vi "Teleop With Vision.vi"(10 "Match Info":T1={"Autonomous Elapsed Seconds"=0.0, "TeleOp Elapsed Seconds"=0.0, "Disabled Elapsed Seconds"=0.0, "Visited Autonomous"=FALSE, "Visited TeleOp"=FALSE, "Visited Disabled"=FALSE, "Autonomous Settings"={"Autonomous Style"=enum."Independent", "VI Refnum"=refnum}}, 11 "Call Context":T2=enum."Execute") -> ()   [LabVIEW 2012]
doc: "This VI is called for each TeleOp packet received from the DS where the robot is not disabled. It is often used to read from the joysticks and update I/O or to update setpoints for timed control loops. It should complete and return within 20 milliseconds or it may miss DS packets."
uses:
  <vilib>/Rock Robotics/WPI/DriverStation/WPI_DriverStationDerivedRobotMode.ctl
  <vilib>/Rock Robotics/WPI/DriverStation/WPI_DriverStationMatch Info.ctl
  Robot Global Data.vi
  <vilib>/Rock Robotics/WPI/RobotDrive/WPI_RobotDriveMecanumDrive_Cartesian.vi
  <vilib>/Rock Robotics/WPI/Joystick/WPI_JoystickGetSetRefNum.vi
  <vilib>/Rock Robotics/WPI/RobotDrive/WPI_RobotDriveGetSetRefNum.vi
panel:
  in  "Rotation Mult":dbl=0.8
  in  "Joystick Mult Slow":dbl=0.5
  in  "Joystick Mult":dbl=1.0
  in  "Rest Speed r/s":dbl=15.0 min=0.0 max=0.7 step=0.05
  out "Angle":dbl(knob)=359.9532640347576 scale=0.0..360.0
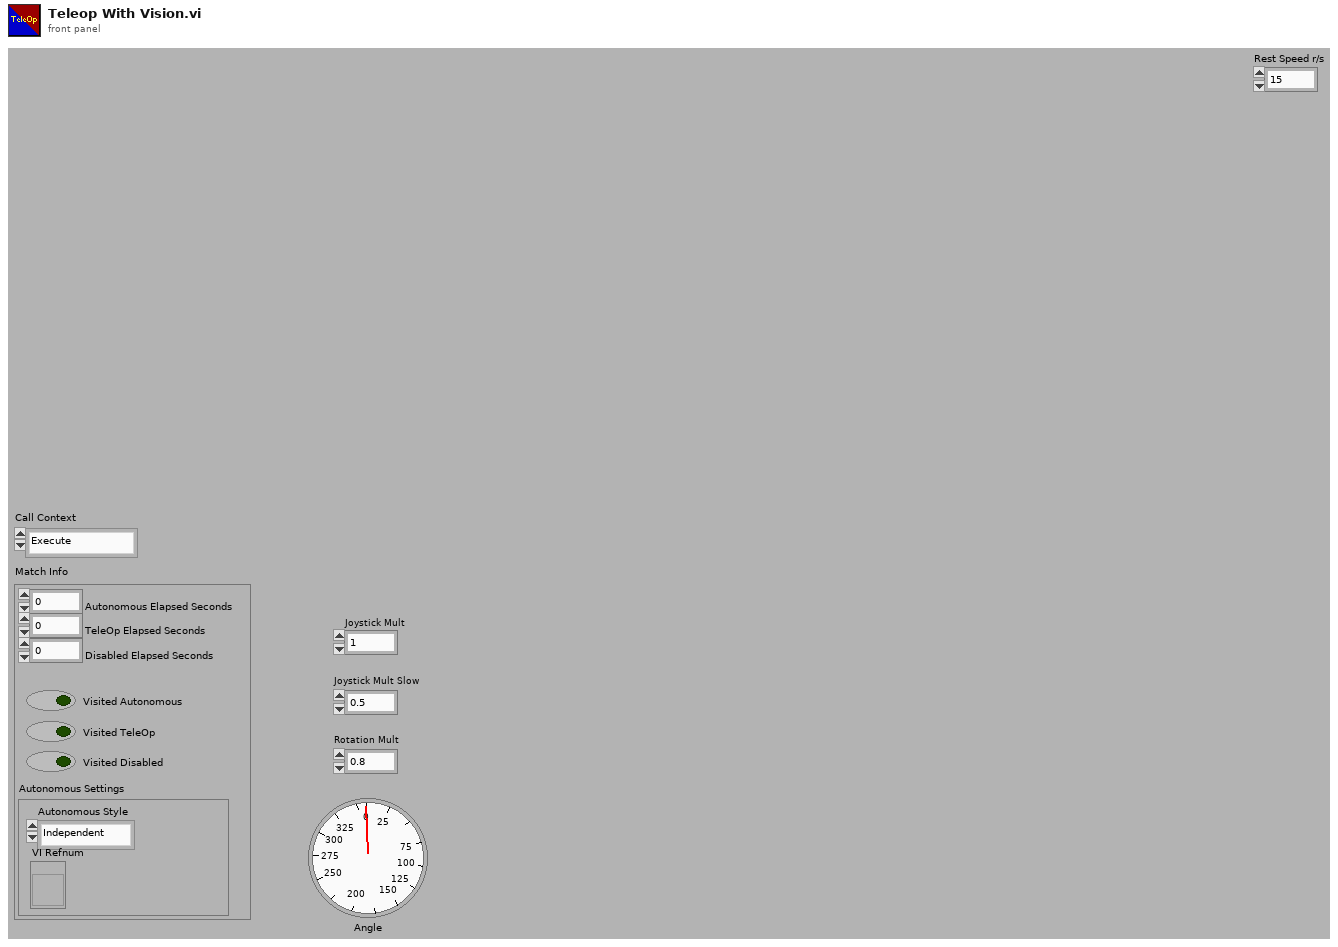
[diagram p1: front panel]
types:
  T1 = typedef "WPI_DriverStationMatch Info.ctl" = cluster{"Autonomous Elapsed Seconds":dbl, "TeleOp Elapsed Seconds":dbl, "Disabled Elapsed Seconds":dbl, "Visited Autonomous":bool, "Visited TeleOp":bool, "Visited Disabled":bool, "Autonomous Settings":cluster{"Autonomous Style":enum16{"Iterative", "Independent"}, "VI Refnum":refnum<vi>}}
  T2 = typedef "WPI_DriverStationDerivedRobotMode.ctl" = enum16{"Init", "Execute", "Stop"}
  T3 = typedef "WPI_JoystickDevRef.ctl" = cluster{"Device":T4}
  T4 = typedef "WPI_JoystickDeviceEnum.ctl" = enum16{"USB 1", "USB 2", "USB 3", "USB 4", "Kinect 1", "Kinect 2"}
  T5 = typedef "WPI_JoystickButtonState.ctl" = cluster{"Button 1":bool, "Button 2":bool, "Button 3":bool, "Button 4":bool, "Button 5":bool, "Button 6":bool, "Button 7":bool, "Button 8":bool, "Button 9":bool, "Button 10":bool, "Button 11":bool, "Button 12":bool}
  T6 = cluster{"axis 1 (x)":dbl, "axis 2 (y)":dbl, "axis 3 (throttle)":dbl, "axis 4":dbl, "axis 5":dbl, "axis 6":dbl}
  T7 = typedef "WPI_GyroDevRef.ctl" = cluster{"DevStatus":errorcluster, "Analog Module":T8, "Analog Channel":T9, "Offset":dbl, "Gain (VoltsPerDegree/Second)":dbl}
  T8 = typedef "FPGA_TypedefAnalogModule.ctl" = enum16{"Analog Module 1", "Analog Module 2"}
  T9 = typedef "FPGA_AIChannel.ctl" = enum8{"AI 1", "AI 2", "AI 3", "AI 4", "AI 5", "AI 6", "AI 7", "AI 8", "Invalid"}
  T10 = typedef "WPI_RobotDriveDevRef.ctl" = cluster{"DevStatus":errorcluster, "Motors[]":T11[], "Square Inputs":bool, "Max Output":dbl, "Isochronous":bool}
  T11 = typedef "WPI_MotorControlDeviceRef.ctl" = cluster{"DeviceStatus":errorcluster, "Type":enum16{"PWM", "CAN"}, "PWM":cluster{"Digital Module":T12, "PWM Channel":T13, "DeadBand":T14}, "CAN":cluster{"Device Number":u8, "Control Mode":T15, "Semaphore":T16, "Max Vout":dbl}, "Invert":bool, "TransformRef":T17, "InvTransformRef":T17}
  T12 = typedef "FPGA_TypedefDigitalModule.ctl" = enum16{"Digital Module 1", "Digital Module 2"}
  T13 = typedef "FPGA_DIOPWMChannel.ctl" = enum8{"PWM 1", "PWM 2", "PWM 3", "PWM 4", "PWM 5", "PWM 6", "PWM 7", "PWM 8", "PWM 9", "PWM 10", "Invalid"}
  T14 = typedef "WPI_PWMDeadband.ctl" = cluster{"Name":string, "maxPositivePwm":i32, "minPositivePwm":i32, "centerPwm":i32, "maxNegativePwm":i32, "minNegativePwm":i32, "angularRange":u16}
  T15 = typedef "WPI_CANJaguar_ControlMode.ctl" = enum8{"Percent VBus", "Current", "Speed", "Position", "Voltage"}
  T16 = typedef "Semaphore RefNum" = refnum<k1>
  T17 = typedef "WPI_PWMTransform_ConPane.ctl" = refnum<vi>
  T18 = typedef "WPI_DigitalInputDevRef.ctl" = cluster{"DevStatus":errorcluster, "DIO Channel":T19, "Digital Module":T12}
  T19 = typedef "FPGA_DIOChannel.ctl" = enum8{"DIO 1", "DIO 2", "DIO 3", "DIO 4", "DIO 5", "DIO 6", "DIO 7", "DIO 8", "DIO 9", "DIO 10", "DIO 11", "DIO 12", "DIO 13", "DIO 14", "Invalid"}
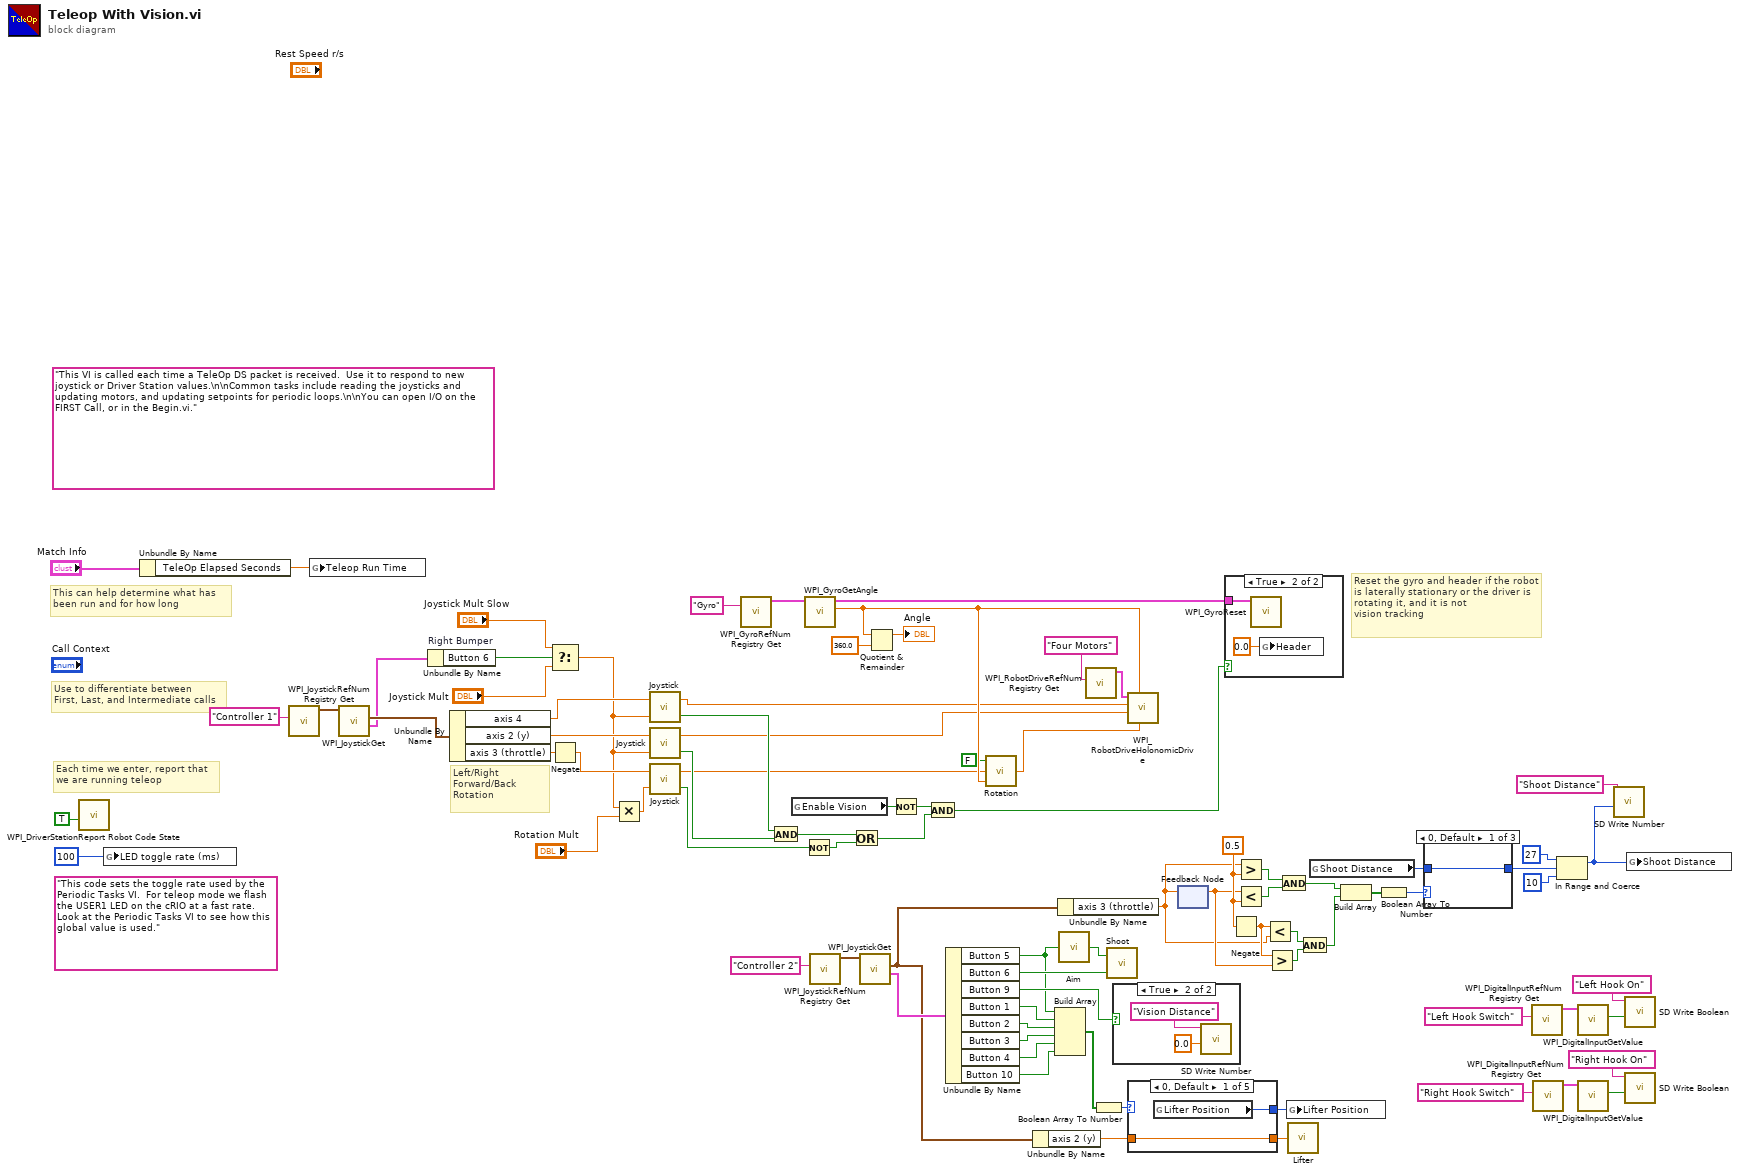
[diagram p0: block diagram]
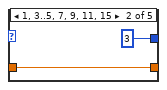
[diagram p2: hidden frame]
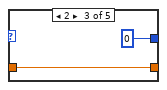
[diagram p3: hidden frame]
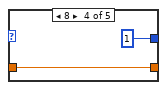
[diagram p4: hidden frame]
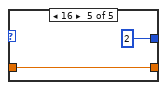
[diagram p5: hidden frame]
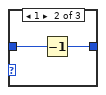
[diagram p6: hidden frame]
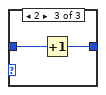
[diagram p7: hidden frame]
diagram:
  w57 = 0.5 ("y")
  (unwired) "This code sets the toggle rate used by the Periodic Tasks VI.  For teleop mode we flash the USER1 LED on the cRIO at a fast rate.  Look at the Periodic Tasks VI to see how this global value is used."
  (unwired) "This VI is called each time a TeleOp DS packet is received.  Use it to respond to new joystick or Driver Station values.\n\nCommon tasks include reading the joysticks and updating motors, and updating setpoints for periodic loops.\n\nYou can open I/O on the FIRST Call, or in the Begin.vi."
  # "Reset the gyro and header if the robot is laterally stationary or the driver is rotating it, and it is not\nvision tracking"
  # "Left/Right\nForward/Back\nRotation"
  # "Each time we enter, report that\nwe are running teleop"
  # "Use to differentiate between\nFirst, Last, and Intermediate calls"
  # "This can help determine what has\nbeen run and for how long"
  n1 = call <vilib>:"WPI_DriverStationReport Robot Code State.vi"("TeleOp"=TRUE ("Autonomous")) -> ()  [unwired: 10 in, 1 out]
  n2 = global write "Robot Global Data.vi" "LED toggle rate (ms)"(u32 100 ("LED ms toggle rate")) -> ()
  n3 = Unbundle By Name("Match Info") -> ("TeleOp Elapsed Seconds"=w25:dbl)
  n4 = call <vilib>:"WPI_JoystickRefNum Registry Get.vi"("refnum name"="Controller 1") -> ("JoystickDevRef"=w82:T3)  [unwired: 1 in, 9 out]
  n5 = global write "Robot Global Data.vi" "Teleop Run Time"(w25) -> ()
  n6 = call <vilib>:"WPI_JoystickGet.vi"("JoystickDevRef"=w82) -> ("Buttons"=w70:T5, "Axes"=w79:T6)  [unwired: 1 in, 4 out]
  n7 = Unbundle By Name "Right Bumper"(w70) -> ("Button 6"=w78:bool)
  n8 = Unbundle By Name(w79) -> ("axis 4"=w21:dbl, "axis 2 (y)"=w20:dbl, "axis 3 (throttle)"=w77:dbl)
  n9 = Select(t="Joystick Mult Slow", s=w78, f="Joystick Mult") -> (s? t:f=w11:dbl)
  n10 = Negate(x=w77) -> (-x=w19:dbl)
  n11 = Multiply(x=w11, y="Rotation Mult") -> (x*y=w12:dbl)
  n12 = call "Joystick.vi"("Multiplier"=w11, "Input"=w21) -> ("In Dead Zone"=w16:bool, "Output"=w15:dbl)
  n13 = call "Joystick.vi"("Multiplier"=w11, "Input"=w20) -> ("In Dead Zone"=w17:bool, "Output"=w14:dbl)
  n14 = call "Joystick.vi"("Multiplier"=w12, "Input"=w19) -> ("In Dead Zone"=w18:bool, "Output"=w13:dbl)
  n15 = call <vilib>:"WPI_GyroRefNum Registry Get.vi"("refnum name"="Gyro") -> ("GyroDevRef"=w76:T7)  [unwired: 9 in, 1 out]
  n16 = And(x=w16, y=w17) -> (x .and. y?=w71:bool)
  n17 = global read "Robot Global Data.vi" "Enable Vision"() -> (w48:bool)
  n18 = Not(x=w18) -> (.not. x?=w44:bool)
  n19 = call <vilib>:"WPI_GyroGetAngle.vi"("GyroDevRef"=w76) -> ("Angle"=w45:dbl, "GyroDevRef"=w75:T7)  [unwired: 7 in, 2 out]
  n20 = call <vilib>:"WPI_JoystickRefNum Registry Get.vi"("refnum name"="Controller 2") -> ("JoystickDevRef"=w66:T3)  [unwired: 1 in, 9 out]
  n21 = Or(x=w71, y=w44) -> (x .or. y?=w65:bool)
  n22 = call <vilib>:"WPI_JoystickGet.vi"("JoystickDevRef"=w66) -> ("Buttons"=w64:T5, "Axes"=w34:T6)  [unwired: 1 in, 4 out]
  n23 = Quotient & Remainder(x=w45, y=360.0) -> (x-y*floor(x/y)=→"Angle":dbl)  [unwired: 1 out]
  n24 = Not(x=w48) -> (.not. x?=w47:bool)
  n25 = And(x=w47, y=w65) -> (x .and. y?=w49:bool)
  n26 = Unbundle By Name(w64) -> ("Button 5"=w28:bool, "Button 6"=w63:bool, "Button 9"=w62:bool, "Button 1"=w43:bool, "Button 2"=w42:bool, "Button 3"=w29:bool, "Button 4"=w41:bool, "Button 10"=w24:bool)
  n27 = call "Rotation.vi"("Gyro Angle"=w45, "Uncorrected Speed"=w13, "Use Correction"=FALSE) -> ("Output Speed"=w68:dbl)
  n28 = Unbundle By Name(w34) -> ("axis 2 (y)"=w32:dbl)
  n29 = Build Array(w28, w43, w42, w29, w41, w24) -> (w40:bool[])
  n30 = Unbundle By Name(w34) -> ("axis 3 (throttle)"=w51:dbl)
  n31 = call "Aim.vi"("Aim"=w28) -> ("Ready"=w46:bool)
  n32 = call <vilib>:"WPI_RobotDriveRefNum Registry Get.vi"("refnum name"="Four Motors") -> ("RobotDriveDevRef"=w69:T10)  [unwired: 1 in, 9 out]
  n33 = Boolean Array To Number(Boolean array=w40) -> (number=w39:u32)
  n34 = call "Shoot.vi"("Shoot"=w63, "Aiming"=w46) -> ()  [unwired: 1 out]
  n35 = case shown="True" w62 {
    frame False {
    }
    frame True {
      n36 = call <vilib>:"SD Write Number.vi"("Numeric"=0.0, "Name"="Vision Distance") -> ()  [unwired: 8 in, 2 out]
    }
  }
  n37 = call-poly <vilib>:"WPI_RobotDriveHolonomicDrive.vi"("Rotation"=w68, "Gyro Angle"=w45, "Y"=w14, "X"=w15, "RobotDriveDevRef"=w69) -> ()  [unwired: 4 in, 3 out]
  n38 = case shown="0, Default" w39 {
    tunnel: [w88 3 0 1 2] -> w27
    tunnel: [w87 w89 w91 w93 w95] -> w33
    tunnel: w32 -> [w87 w89 w91 w93 w95]
    frame 0, Default {
      n39 = global read "Robot Global Data.vi" "Lifter Position"() -> (w88:i8)
    }
    frame 1, 3..5, 7, 9, 11, 15 {
    }
    frame 2 {
    }
    frame 8 {
    }
    frame 16 {
    }
  }
  n40 = feedback #1() -> (w55:dbl)  [unwired: 1 in]
  n41 = feedback-in #1(w51) -> ()
  n42 = case shown="True" w49 {
    tunnel: w75 -> [_ w98]
    frame False {
    }
    frame True {
      n43 = call <vilib>:"WPI_GyroReset.vi"("GyroDevRef"=w98) -> ()  [unwired: 11 out]
      n44 = global write "Robot Global Data.vi" "Header"(0.0 ("Header")) -> ()
    }
  }
  n45 = Negate(x=w57) -> (-x=w56:dbl)
  n46 = Greater?(x=w51, y=w57) -> (0:w60:bool)
  n47 = Less?(x=w55, y=w57) -> (x < y?=w61:bool)
  n48 = Less?(x=w56, y=w51) -> (x < y?=w58:bool)
  n49 = Greater?(x=w56, y=w55) -> (0:w59:bool)
  n50 = And(x=w60, y=w61) -> (x .and. y?=w54:bool)
  n51 = global write "Robot Global Data.vi" "Lifter Position"(w27) -> ()
  n52 = call "Lifter.vi"("Custom Speed"=w33) -> ()  [unwired: 1 out]
  n53 = And(x=w58, y=w59) -> (x .and. y?=w53:bool)
  n54 = global read "Robot Global Data.vi" "Shoot Distance"() -> (w38:i32)
  n55 = Build Array(w54, w53) -> (w52:bool[])
  n56 = Boolean Array To Number(Boolean array=w52) -> (number=w50:u32)
  n57 = case shown="0, Default" w50 {
    tunnel: w38 -> [w99 w101 w103]
    tunnel: [w99 w100 w102] -> w37
    frame 0, Default {
    }
    frame 1 {
      n58 = Decrement(x=w101) -> (x-1=w100:i32)
    }
    frame 2 {
      n59 = Increment(x=w103) -> (x+1=w102:i32)
    }
  }
  n60 = call <vilib>:"WPI_DigitalInputRefNum Registry Get.vi"("refnum name"="Left Hook Switch") -> ("DigitalInputDevRef"=w6:T18)  [unwired: 9 in, 1 out]
  n61 = call <vilib>:"WPI_DigitalInputRefNum Registry Get.vi"("refnum name"="Right Hook Switch") -> ("DigitalInputDevRef"=w5:T18)  [unwired: 9 in, 1 out]
  n62 = In Range and Coerce(upper limit=27, x=w37, lower limit=10) -> (coerced(x)=w30:i32)  [unwired: 1 out]
  n63 = call <vilib>:"WPI_DigitalInputGetValue.vi"("DigitalInputDevRef"=w6) -> ("Value"=w4:bool)  [unwired: 8 in, 2 out]
  n64 = call <vilib>:"WPI_DigitalInputGetValue.vi"("DigitalInputDevRef"=w5) -> ("Value"=w3:bool)  [unwired: 8 in, 2 out]
  n65 = call <vilib>:"SD Write Number.vi"("Numeric"=w30, "Name"="Shoot Distance") -> ()  [unwired: 8 in, 2 out]
  n66 = call <vilib>:"SD Write Boolean.vi"("Boolean"=w4, "Name"="Left Hook On") -> ()  [unwired: 8 in, 2 out]
  n67 = call <vilib>:"SD Write Boolean.vi"("Boolean"=w3, "Name"="Right Hook On") -> ()  [unwired: 8 in, 2 out]
  n68 = global write "Robot Global Data.vi" "Shoot Distance"(w30) -> ()
